vi "Configure Measurement Type.vi"(8 "error in (no error)":errorcluster, 9 "Measurement Mode (0: Off)":i32(ring) items=["Off", "Channel Power Measurement", "Adjacent Channel Power Ratio Measurement", "Occupied Bandwidth Measurement", "Spectrum Monitor", "Spectrum Emission Mask", "Channel Scanner", "AM Measurement", "ASK Measurement", "FM Measurement", "FSK Measurement"], 10 "Measurement Type (0: Spectrum Analyzer)":i32(ring) items=["Spectrum Analyzer", "Tracking Generator", "Power Meter", "Modulation Analyzer", "Reflection Measurement"], 11 "VISA resource name":refnum<visa-resource-name>) -> (0 "error out":errorcluster, 3 "VISA resource name out":refnum<visa-resource-name>)   [LabVIEW 2022 SP3, in "Agilent N934X Series.lvlib"]
doc: "Selects the measurement type of the analyzer. Before you perform any measurement, you must call this VI to select the measurement type."
uses:
  <instrlib>/Agilent N934X Series/Agilent N934X Series.lvlib
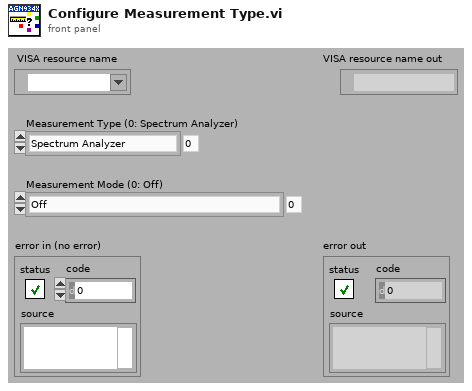
[diagram p1: front panel]
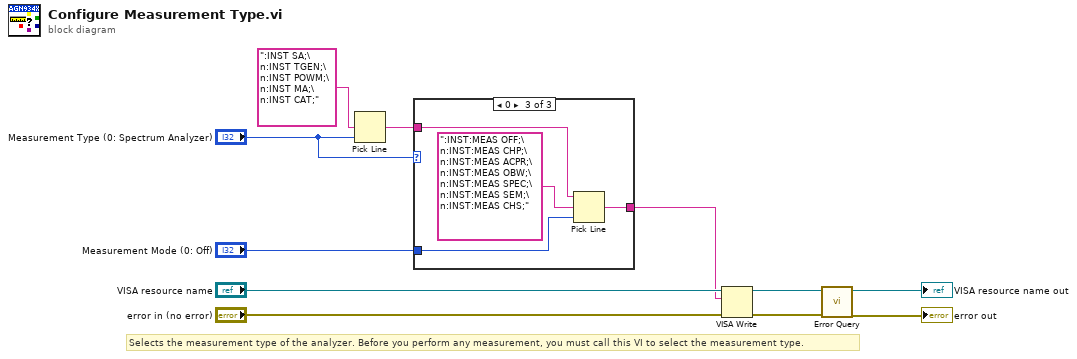
[diagram p0: block diagram]
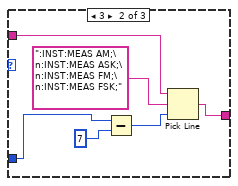
[diagram p3: hidden frame]
diagram:
  # "Selects the measurement type of the analyzer. Before you perform any measurement, you must call this VI to select the measurement type."
  n1 = Pick Line(multi-line string=":INST SA;\n:INST TGEN;\n:INST POWM;\n:INST MA;\n:INST CAT;", line index="Measurement Type (0: Spectrum Analyzer)") -> (output string=w3:string)  [unwired: 1 in]
  n2 = case shown="0" "Measurement Type (0: Spectrum Analyzer)" {
    tunnel: w3 -> [w12 w13 w21]
    tunnel: [w12 w18 w20] -> w2
    tunnel: "Measurement Mode (0: Off)" -> [_ w17 w19]
    frame 1, 2, Default {
    }
    frame 3 {
      n3 = Subtract(x=w17, y=7) -> (x-y=w15:i32)
      n4 = Pick Line(string ("")=w13, multi-line string=":INST:MEAS AM;\n:INST:MEAS ASK;\n:INST:MEAS FM;\n:INST:MEAS FSK;", line index=w15) -> (output string=w18:string)
    }
    frame 0 {
      n5 = Pick Line(string ("")=w21, multi-line string=":INST:MEAS OFF;\n:INST:MEAS CHP;\n:INST:MEAS ACPR;\n:INST:MEAS OBW;\n:INST:MEAS SPEC;\n:INST:MEAS SEM;\n:INST:MEAS CHS;", line index=w19) -> (output string=w20:string)
    }
  }
  n6 = VISA Write(VISA resource name="VISA resource name", write buffer=w2, error in (no error)="error in (no error)") -> (VISA resource name out=w8:refnum<visa-resource-name>, error out=w7:errorcluster)  [unwired: 1 out]
  n7 = call <instrlib>:"Error Query.vi"("error in (no error)"=w7, "VISA resource name"=w8) -> ("error out"=→"error out":errorcluster, "VISA resource name out"=→"VISA resource name out":refnum<visa-resource-name>)  [unwired: 6 in, 2 out]
